vi "create_standardized_delay_array.vi"(3 "burst period":dbl, 4 "delay array":dbl[](array[numeric]), 5 "resolution":i32=100) -> (0 "corrected burst period":dbl, 1 "standardize array":dbl[](array[numeric]), 2 "multiplier":i32)   [LabVIEW 2011]
doc: "creates a standardize array that can be easily displayed no matter what the time unit in the array is. covers second to nanoseconds."
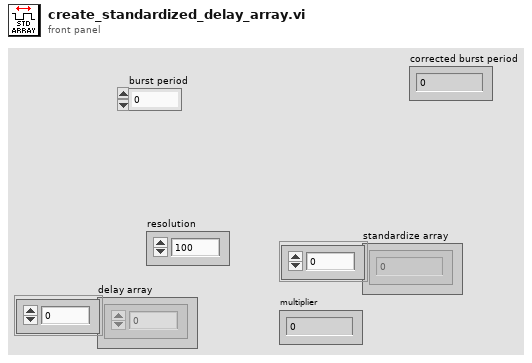
[diagram p1: front panel]
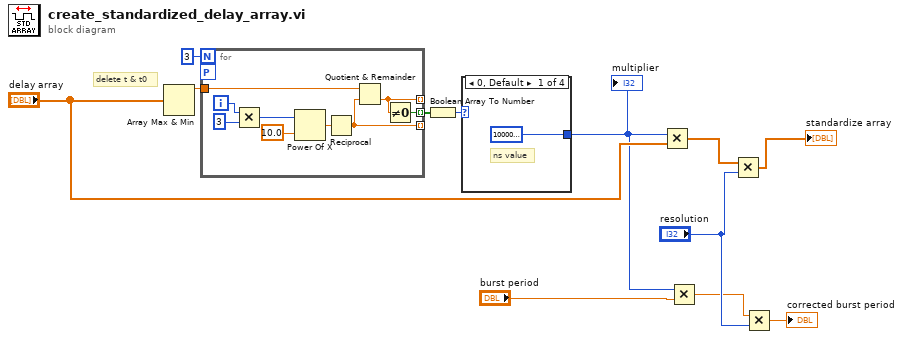
[diagram p0: block diagram]
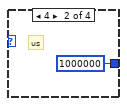
[diagram p2: hidden frame]
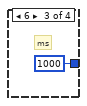
[diagram p3: hidden frame]
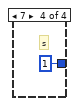
[diagram p4: hidden frame]
diagram:
  # "delete t & t0"
  n1 = Array Max & Min(array="delay array") -> (max value=w9:dbl)  [unwired: 3 out]
  n2 = for {
    N: 3 -> [_]
    tunnel: w9 -> [w18]
    tunnel: [w13] -> _ mode=indexing
    tunnel: [w17] -> _ mode=indexing
    tunnel: [w16] -> w11 mode=indexing
    workers-P: _ -> [_]
    i -> [w15]
    n3 = Multiply(x=w15, y=3) -> (x*y=w19:i32)
    n4 = Power Of X(1:10.0 ("x"), 2:w19) -> (0:w14:dbl)
    n5 = Reciprocal(x=w14) -> (1/x=w13:dbl)
    n6 = Quotient & Remainder(x=w18, y=w13) -> (floor(x/y)=w17:dbl)  [unwired: 1 out]
    n7 = Not Equal To 0?(x=w17) -> (x != 0?=w16:bool)
  }
  n8 = Boolean Array To Number(Boolean array=w11) -> (number=w10:u32)
  n9 = case shown="0, Default" w10 {
    tunnel: [1000000000 1000000 1000 1] -> w4
    frame 0, Default {
      # "ns value"
    }
    frame 4 {
      # "us"
    }
    frame 6 {
      # "ms"
    }
    frame 7 {
      # "s"
    }
  }
  "multiplier" <- w4
  n10 = Multiply(x=w4, y="delay array") -> (x*y=w8:dbl[])
  n11 = Multiply(x=w4, y="burst period") -> (x*y=w2:dbl)
  n12 = Multiply(x=w8, y="resolution") -> (x*y=→"standardize array":dbl[])
  n13 = Multiply(x=w2, y="resolution") -> (x*y=→"corrected burst period":dbl)
